vi "DevToStr.vi"(0 "Device in":refnum<class "Device.lvclass">) -> (2 "Device String":string, 3 "Partial Table Transpose":string[][](array[string]))   [LabVIEW 2013]
uses:
  DeviceVIs/Device/Device.lvclass
  ColumnVIs/Column/Column.lvclass
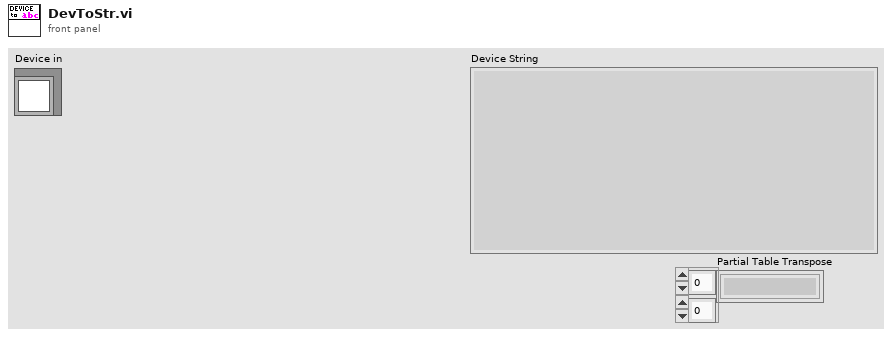
[diagram p1: front panel]
types:
  T1 = typedef "ColumnAppearCluster.ctl" = cluster{"Column Name":string, "Width":u32, "Bkgd":u32[], "Text":u32[]}
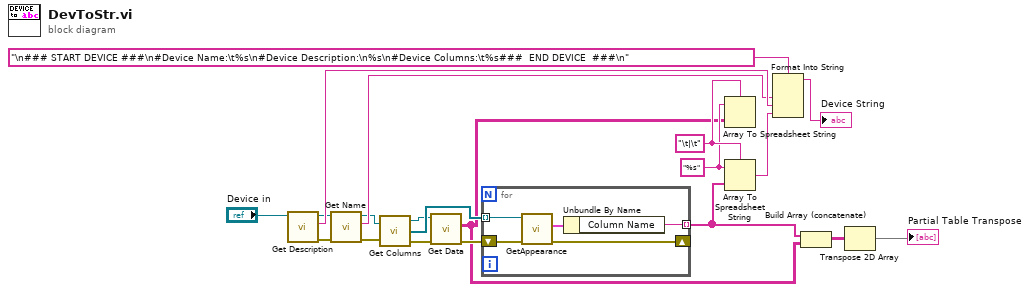
[diagram p0: block diagram]
diagram:
  w5 = "%s" ("format string")
  w6 = "\t|\t" ("format string")
  n1 = call-dynamic "Get Description.vi"("Device in"="Device in") -> ("error out"=w16:errorcluster, "Device Description"=w20:string, "Device out"=w17:refnum<class "Device.lvclass">)  [unwired: 8 in]
  n2 = call-dynamic "Get Name.vi"("error in (no error)"=w16, "Device in"=w17) -> ("error out"=w15:errorcluster, "Name"=w19:string, "Device out"=w14:refnum<class "Device.lvclass">)  [unwired: 7 in]
  n3 = call-dynamic "Get Columns.vi"("Device in"=w14, "error in (no error)"=w15) -> ("Device out"=w10:refnum<class "Device.lvclass">, "Columns"=w13:refnum<class "Column.lvclass">[], "error out"=w9:errorcluster)
  n4 = call-dynamic "Get Data.vi"("error in (no error)"=w9, "Device in"=w10) -> ("error out"=w8:errorcluster, "Table Indicator"=w4:string[][])  [unwired: 6 in, 1 out]
  n5 = for {
    tunnel: w13 -> [w25] mode=indexing
    tunnel: [w21] -> w3 mode=indexing
    shift-right: [w24] -> _
    shift-left: w8 -> [w23]
    n6 = call "GetAppearance.vi"("error in (no error)"=w23, "Column in"=w25) -> ("error out"=w24:errorcluster, "Column Appearance"=w22:T1)  [unwired: 7 in, 1 out]
    n7 = Unbundle By Name(w22) -> ("Column Name"=w21:string)
  }
  n8 = Array To Spreadsheet String(delimiter (Tab)=w6, array=w4, 3:w5) -> ()  [unwired: 1 out]
  n9 = Array To Spreadsheet String(delimiter (Tab)=w6, array=w3, 3:w5) -> (spreadsheet string=w7:string)
  n10 = Format Into String(format string="\n### START DEVICE ###\n#Device Name:\t%s\n#Device Description:\n%s\n#Device Columns:\t%s###  END DEVICE  ###\n", w19, w20, w7) -> (resulting string=→"Device String":string)  [unwired: 2 in, 1 out]
  n11 = Build Array (concatenate)(w3, w4) -> (w2:string[][])
  n12 = Transpose 2D Array(2D array=w2) -> (transposed array=→"Partial Table Transpose":string[][])
